vi "LED Matrix Send.vi"(5 "Gamma":dbl=2.5, 7 "error in (no error)":errorcluster, 8 "Brightness":u8=50 max=100 step=1, 9 "Data":u32[](array[numeric]), 10 "Refnum in":refnum<k20>) -> (0 "error out":errorcluster, 3 "Refnum out":refnum<k20>, 4 "LED Matrix":picture)   [LabVIEW 2013]
uses:
  <vilib>/picture/picture.llb/imagedata.ctl
  <vilib>/rvi/interface/common/niFpgaWaitOnOcc.vi
  <vilib>/Utility/error.llb/Error Cluster From Error Code.vi
  <vilib>/rvi/errors/niLvFpgaAdjustHostInterfaceError.vi
  <vilib>/rvi/interface/nirviReadWriteControl/nirviReadWriteControl.xnode
  NiFpgaLv.dll
  <vilib>/rvi/interface/Simulation/niFpgaSimulationCallBeginRW.vi
panel:
  in  "Width":i16=32
  in  "Height":i16=16
  # "For now, leave Height & Width as internal constants.\nHowever, it would be trivial to make them controls."
  # "Would like to be able to output a picture that\nlooks the same as what the LED Matrix is displaying\nbut this feature is not yet working. So do not add\nit to a terminal yet."
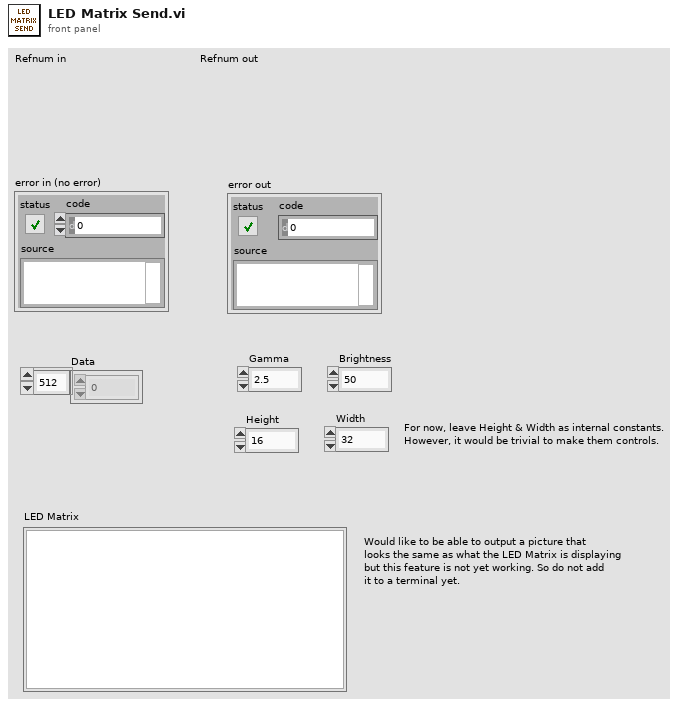
[diagram p1: front panel]
types:
  T1 = typedef "imagedata.ctl" = cluster{"image type":i32, "image depth":i32, "image":u8[], "mask":u8[], "colors":u32[], "Rectangle":cluster{"left":i16, "top":i16, "right":i16, "bottom":i16}}
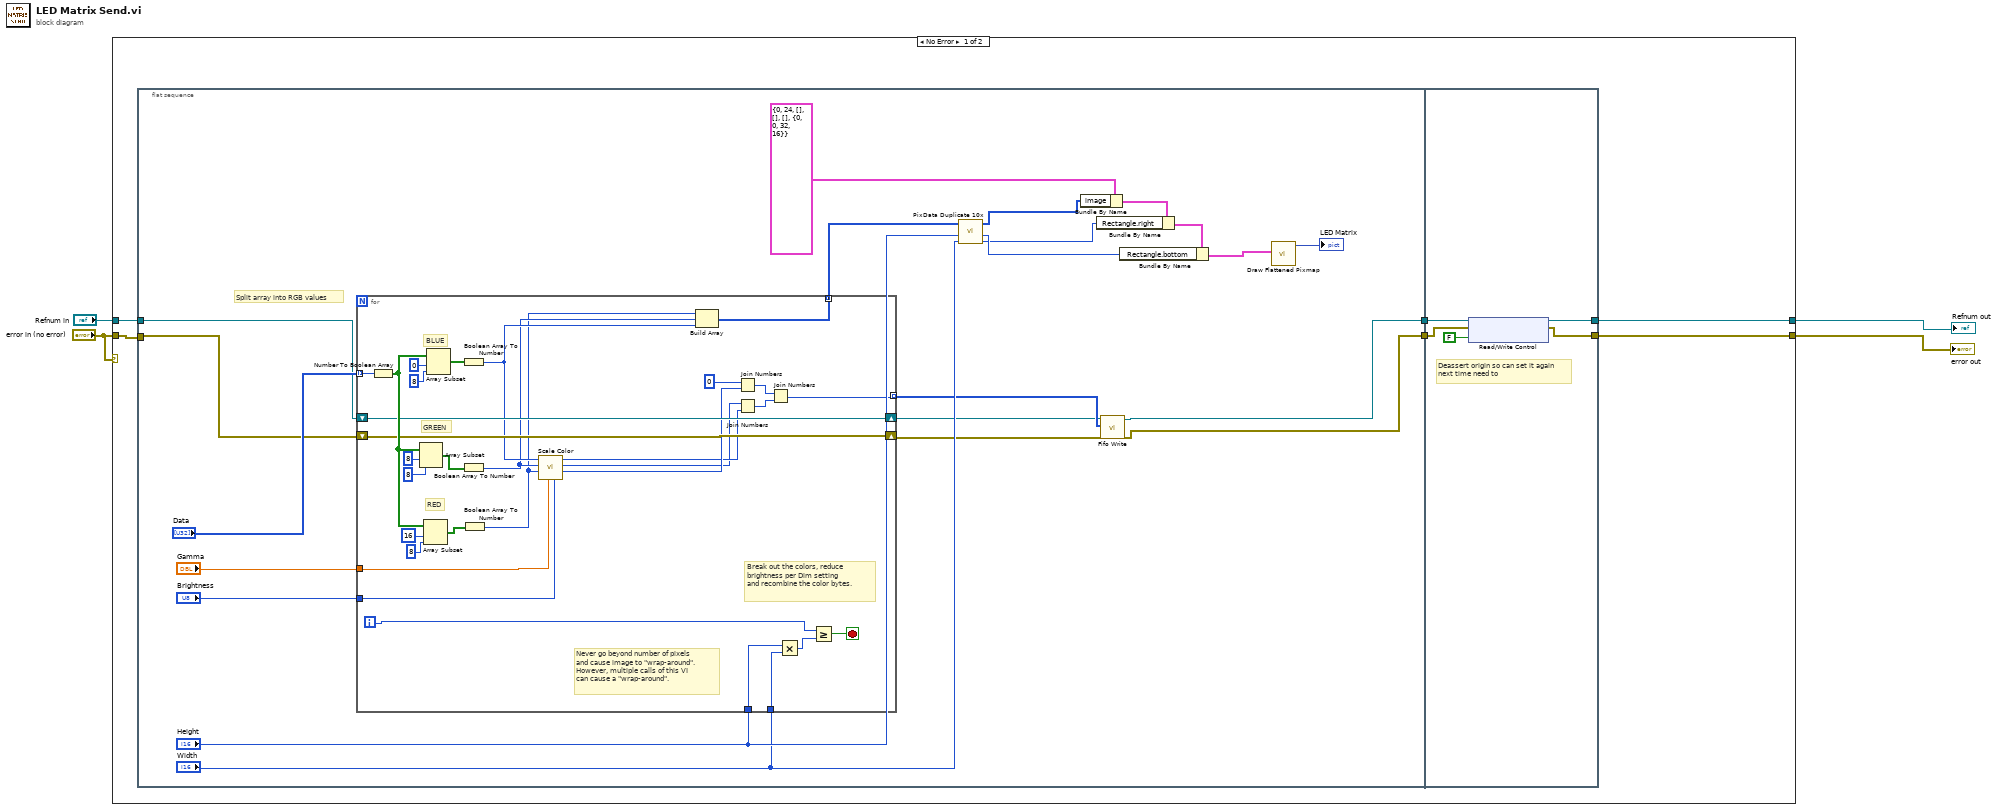
[diagram p0: block diagram]
diagram:
  n1 = case shown="No Error" "error in (no error)" {
    tunnel: [w9 w69] -> w4
    tunnel: "error in (no error)" -> [w5 w68]
    tunnel: "Refnum in" -> [w6 w69]
    tunnel: [w10 w68] -> w2
    frame No Error {
      n2 = flat-sequence {
        tunnel: [w15] -> w8
        tunnel: [w16] -> w7
        tunnel: w6 -> [w30]
        tunnel: w5 -> [w29]
        tunnel: [w66] -> w9
        tunnel: [w63] -> w10
        tunnel: w8 -> [w64]
        tunnel: w7 -> [w65]
        frame #0 {
          # "Split array into RGB values"
          n3 = for {
            tunnel: "Data" -> [w62] mode=indexing
            shift-right: [w42] -> w13
            shift-left: w30 -> [w42]
            shift-right: [w41] -> w14
            shift-left: w29 -> [w41]
            tunnel: [w45] -> w22 mode=concatenating
            tunnel: "Height" -> [w44]
            tunnel: "Width" -> [w43]
            tunnel: [w40] -> w17 mode=indexing
            tunnel: "Gamma" -> [w35]
            tunnel: "Brightness" -> [w36]
            i -> [w47]
            stop <- w48 stop-if-true
            # "BLUE"
            # "GREEN"
            # "RED"
            # "Never go beyond number of pixels\nand cause image to \"wrap-around\".\nHowever, multiple calls of this VI \ncan cause a \"wrap-around\"."
            # "Break out the colors, reduce brightness per Dim setting\nand recombine the color bytes."
            n4 = Number To Boolean Array(number=w62) -> (Boolean array=w52:bool[])
            n5 = Array Subset(array=w52, index=8, length=8) -> (w54:bool[])
            n6 = Array Subset(array=w52, index=16, length=8) -> (w53:bool[])
            n7 = Array Subset(array=w52, index=0, length=8) -> (w55:bool[])
            n8 = Boolean Array To Number(Boolean array=w55) -> (number=w38:u8)
            n9 = Boolean Array To Number(Boolean array=w54) -> (number=w37:u8)
            n10 = Boolean Array To Number(Boolean array=w53) -> (number=w34:u8)
            n11 = call "Scale Color.vi"("Brightness"=w36, "Factor"=w35, "Red"=w34, "Green"=w37, "Blue"=w38) -> ("Red Out"=w39:u8, "Green Out"=w32:u8, "Blue Out"=w33:u8)  [unwired: 4 in]
            n12 = Build Array(w34, w37, w38) -> (w45:u8[])
            n13 = Join Numbers(hi=w32, lo=w33) -> ((hi.lo)=w50:u16)
            n14 = Join Numbers(hi=u8 0, lo=w39) -> ((hi.lo)=w49:u16)
            n15 = Join Numbers(hi=w49, lo=w50) -> ((hi.lo)=w40:u32)
            n16 = Multiply(x=w44, y=w43) -> (x*y=w46:i16)
            n17 = Greater Or Equal?(x=w47, y=w46) -> (x >= y?=w48:bool)
          }
          n18 = call "PixData Duplicate 10x.vi"("Width"="Width", "Height"="Height", "PixData In"=w22) -> ("Output Width"=w18:i16, "Output Height"=w19:i16, "PixData Out"=w23:u8[])  [unwired: 6 in]
          n19 = Bundle By Name(cluster=T1 {"image type"=0, "image depth"=24, "image"=[], "mask"=[], "colors"=[], "Rectangle"={"left"=0, "top"=0, "right"=32, "bottom"=16}} ("image data"), "image"=w23) -> (w26:T1)
          n20 = Bundle By Name(cluster=w26, "Rectangle.right"=w18) -> (w25:T1)
          n21 = call "Fifo Write.vi"("error in (no error)"=w14, "Data"=w17, "Refnum in"=w13) -> ("error out"=w15:errorcluster, "Refnum out"=w16:refnum<k20>)  [unwired: 7 in]
          n22 = Bundle By Name(cluster=w25, "Rectangle.bottom"=w19) -> (w24:T1)
          n23 = call <vilib>:"Draw Flattened Pixmap.vi"("image data"=w24) -> ("new picture"=→"LED Matrix":picture)  [unwired: 8 in]
        }
        frame #1 {
          # "Deassert origin so can set it again\nnext time need to"
          n24 = xnode "Read/Write Control"("FPGA VI Reference In"=w65, "error in"=w64, "LEDMatrix.origin"=FALSE) -> ("FPGA VI Reference Out"=w66:refnum<k20>, "error out"=w63:errorcluster)
        }
      }
    }
    frame Error {
    }
  }
  "Refnum out" <- w4
  "error out" <- w2
